vi "REDXdll.vi"(8 "error in (no error)":errorcluster, 9 "D":dbl, 10 "t":dbl, 11 "z":dbl[](array[numeric])) -> (0 "error out":errorcluster, 1 "D out":dbl, 2 "t out":dbl, 3 "z out":dbl[](array[numeric]))   [LabVIEW 2016]
doc: "subroutine REDXdll(z, t, D)\n\nReturns the reducing parameters associated with mixture EOS; used to calculate the ‘tau’ and ‘del’, which are\nthe independent variables in the EOS.\n\nINPUTS:\nz --Composition (array of mole fractions)\nt--temperature [K] \nD--overall (bulk) molar density [mol/L]"
uses:
  REFPROP.DLL
panel:
  # "REFPROP- REDXdll.vi"
  # "void  REDXdll(double *z, double *t, double *D)"
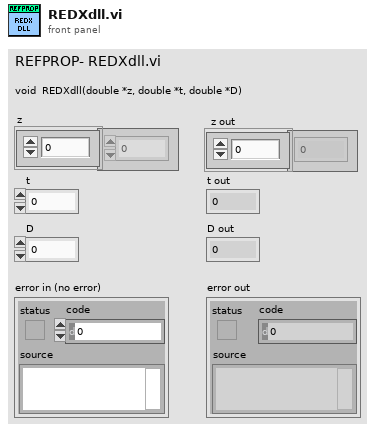
[diagram p1: front panel]
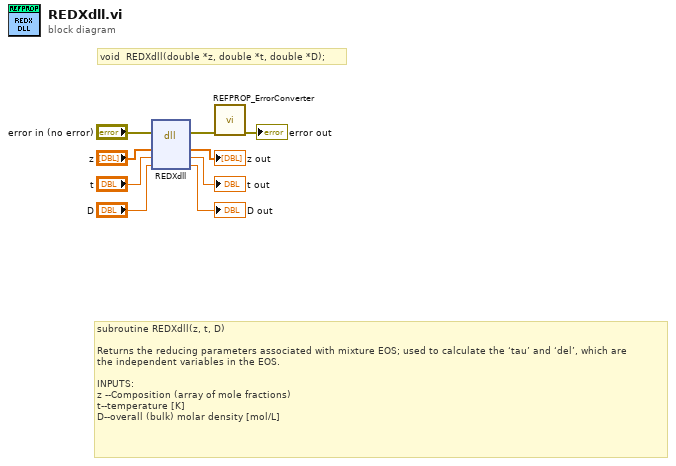
[diagram p0: block diagram]
diagram:
  # "void  REDXdll(double *z, double *t, double *D);"
  # "subroutine REDXdll(z, t, D)\n\nReturns the reducing parameters associated with mixture EOS; used to calculate the ‘tau’ and ‘del’, which are\nthe independent variables in the EOS.\n\nINPUTS:\nz --Composition (array of mole fractions)\nt--temperature [K] \nD--overall (bulk) molar density [mol/L]"
  n1 = dll-call lib="S:/009 - Testing/02 - Performance Testing/REFPROP/REFPROP.*" fn="REDXdll"(error in="error in (no error)", "z"="z", "t"="t", "D"="D") -> (error out=w3:errorcluster, "z"=→"z out":dbl[], "t"=→"t out":dbl, "D"=→"D out":dbl)  [unwired: 3 in, 1 out]
  n2 = call "REFPROP_ErrorConverter.vi"("error in (no error)"=w3) -> ("error out"=→"error out":errorcluster)  [unwired: 10 in]
